vi "USBTC08errorhandler.vi"(7 "Close unit":bool, 8 "error in (no error)":errorcluster, 9 "Return":i16, 10 "API function":string, 11 "Handle in":i16) -> (0 "error out":errorcluster, 3 "Handle out":i16)   [LabVIEW 2009]
uses:
  usbtc08.dll
panel:
  out "stop unit return type":i16
  out "close_unit return type":i16
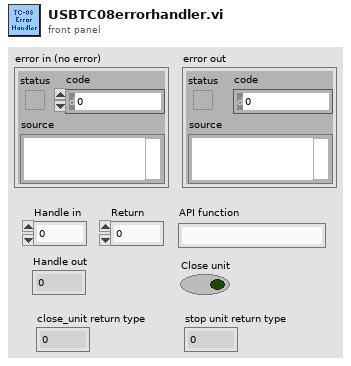
[diagram p1: front panel]
types:
  T1 = enum16{"Left Button", "Center Button", "Right Button", "Window Close"}
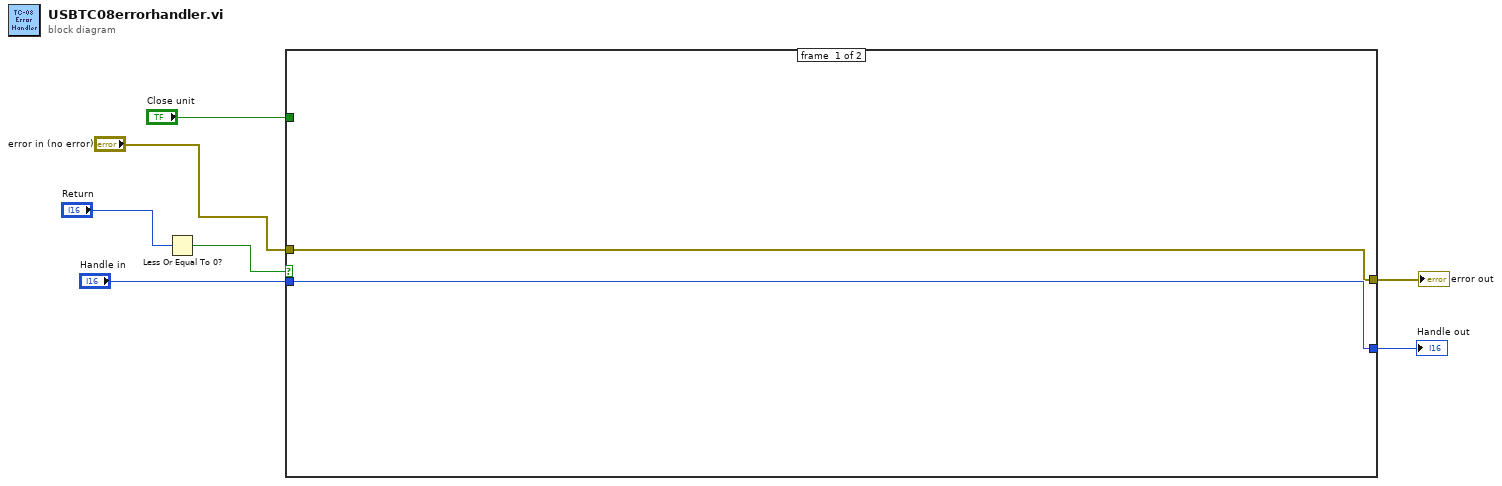
[diagram p0: block diagram]
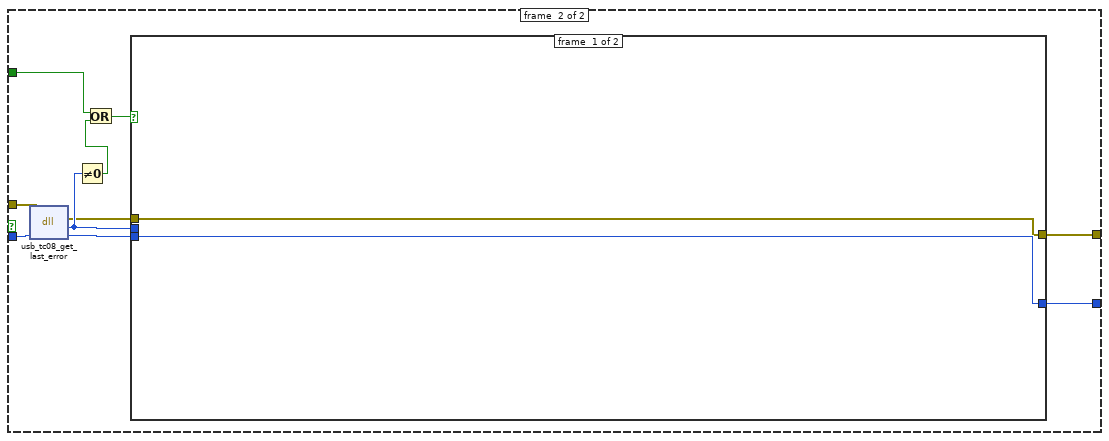
[diagram p2: hidden frame]
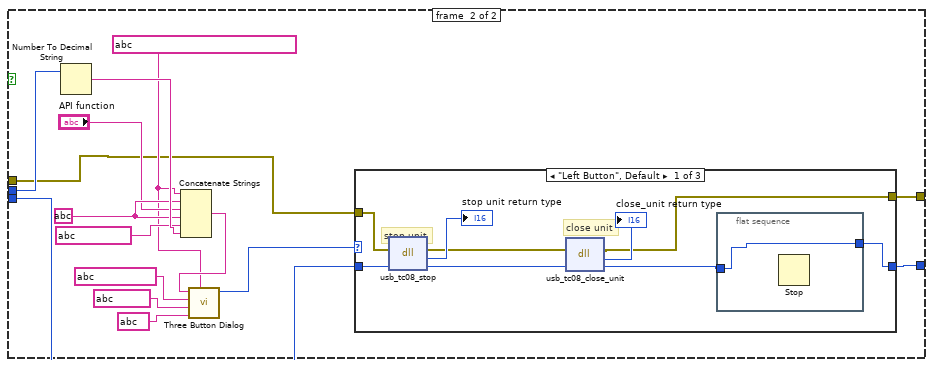
[diagram p3: hidden frame]
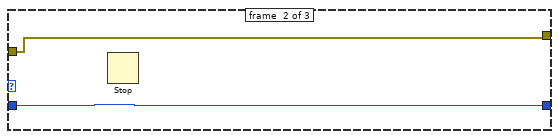
[diagram p4: hidden frame]
diagram:
  n1 = Less Or Equal To 0?(x="Return") -> (x <= 0?=w5:bool)
  n2 = case shown="True" w5 {
    tunnel: "Handle in" -> [w9 w19]
    tunnel: [w9 w17] -> w4
    tunnel: "error in (no error)" -> [w8 w15]
    tunnel: [w8 w13] -> w2
    tunnel: "Close unit" -> [_ w12]
    frame #0 {
    }
    frame #1 {
      n3 = dll-call lib="usbtc08.dll" fn="usb_tc08_get_last_error" label="get_last_error"(error in=w15, "Handle"=w19) -> (error out=w14:errorcluster, "Return"=w16:i16, "Handle"=w18:i16)  [unwired: 2 in, 1 out]
      n4 = Not Equal To 0?(x=w16) -> (x != 0?=w11:bool)
      n5 = Or(x=w12, y=w11) -> (x .or. y?=w10:bool)
      n6 = case shown="True" w10 {
        tunnel: w18 -> [w21 w32]
        tunnel: w16 -> [_ w31]
        tunnel: [w21 w24] -> w17
        tunnel: w14 -> [w20 w23]
        tunnel: [w20 w22] -> w13
        frame #0 {
        }
        frame #1 {
          w27 = string ?
          w25 = string ?
          n7 = Number To Decimal String(number=w31) -> (decimal integer string=w29:string)  [unwired: 1 in]
          n8 = Concatenate Strings(w25, w27, "API function", w27, string ? ("string"), w29) -> (w30:string)
          n9 = call <vilib>:"Three Button Dialog.vi"("Window Title (\"\")"=w25, "Right Button Text (\"Cancel\")"=string ? ("Right Button Text (\"Cancel\")"), "Center Button Text (\"No\")"=string ? ("Center Button Text (\"No\")"), "Left Button Text (\"Yes\")"=string ? ("Left Button Text (\"Yes\")"), "message"=w30) -> ("Which Button?"=w33:T1)  [unwired: 6 in]
          n10 = case shown="\"Left Button\", Default" w33 {
            tunnel: w32 -> [w44 w48 w50]
            tunnel: [w40 w48 w50] -> w24
            tunnel: w23 -> [w39 w47 w49]
            tunnel: [w37 w47 w49] -> w22
            frame #0 {
              # "close unit"
              # "stop unit"
              n11 = dll-call lib="usbtc08.dll" fn="usb_tc08_stop" ("Close unit")(error in=w39, "handle"=w44) -> (error out=w38:errorcluster, "return type"=→"stop unit return type":i16, "handle"=w45:i16)  [unwired: 2 in, 1 out]
              n12 = dll-call lib="usbtc08.dll" fn="usb_tc08_close_unit" ("Close unit")(error in=w38, "handle"=w45) -> (error out=w37:errorcluster, "return type"=→"close_unit return type":i16, "handle"=w41:i16)  [unwired: 2 in, 1 out]
              n13 = flat-sequence {
                tunnel: w41 -> [w46]
                tunnel: [w46] -> w40
                frame #0 {
                  n14 = Stop() -> ()  [unwired: 1 in]
                }
              }
            }
            frame #1 {
              n15 = Stop() -> ()  [unwired: 1 in]
            }
            frame #2 {
            }
          }
        }
      }
    }
  }
  "Handle out" <- w4
  "error out" <- w2
